vi "ModelParameters.SetModelParameterValue.vi"(8 "Value to Set":dbl, 9 "Channel Name":string, 10 "Target Name":string, 11 "GatewayIP":string) -> (0 "error out":errorcluster)   [LabVIEW 2013, in "MiscHelperVIs.lvlib"]
uses:
  MiscHelperVIs.lvlib
  <vilib>/NI Veristand/Execution/ModelManager/NI VeriStand - Set Single Parameter Value.vi
  <vilib>/NI Veristand/Execution/ModelManager/NI VeriStand - Get Single Parameter Value.vi
  <vilib>/NI Veristand/Execution/ModelManager/NI_VS ModelManager ExecutionAPI.lvlib
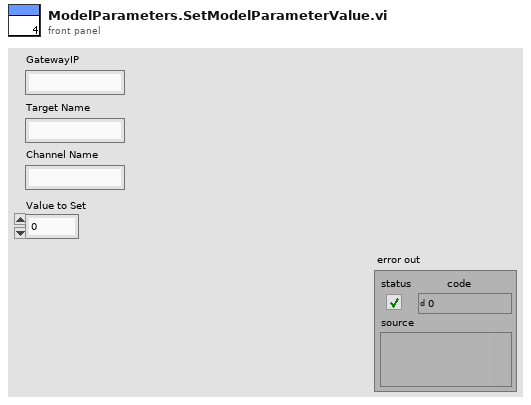
[diagram p1: front panel]
types:
  T1 = typedef "NI_VS ModelManager ExecutionAPI.lvlib/ModelManagerAPI.ctl" = refnum<k24>
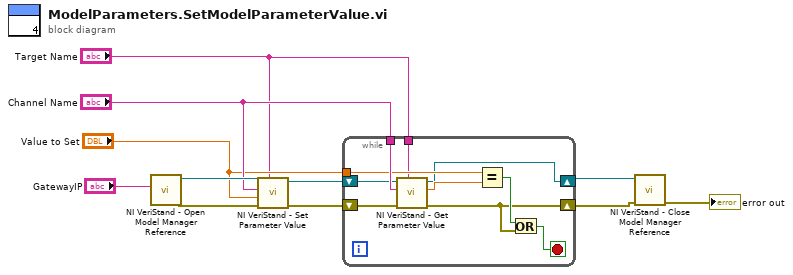
[diagram p0: block diagram]
diagram:
  n1 = call <vilib>:"NI VeriStand - Open Model Manager Reference.vi"("Gateway IP Address (\"\": localhost)"="GatewayIP") -> ("error out"=w10:errorcluster, "ModelManager"=w9:T1)  [unwired: 9 in]
  n2 = call-poly <vilib>:"NI VeriStand - Set Parameter Value.vi"("Target"="Target Name", "error in (no error)"=w10, "Value"="Value to Set", "Parameter"="Channel Name", "ModelManager in"=w9) -> ("error out"=w5:errorcluster, "ModelManager out"=w4:T1)  [unwired: 5 in]
  n3 = while {
    tunnel: "Channel Name" -> [w21]
    tunnel: "Value to Set" -> [w19]
    shift-right: [w14] -> w2
    shift-left: w4 -> [w17]
    tunnel: "Target Name" -> [w13]
    shift-right: [w12] -> w1
    shift-left: w5 -> [w18]
    stop <- w15 stop-if-true
    n4 = call-poly <vilib>:"NI VeriStand - Get Parameter Value.vi"("Target"=w13, "error in (no error)"=w18, "Parameter"=w21, "ModelManager in"=w17) -> ("error out"=w12:errorcluster, "Value"=w20:dbl, "ModelManager out"=w14:T1)  [unwired: 5 in]
    n5 = Equal?(x=w19, y=w20) -> (x = y?=w16:bool)
    n6 = Or(x=w16, y=w12) -> (x .or. y?=w15:bool)
  }
  n7 = call <vilib>:"NI VeriStand - Close Model Manager Reference.vi"("error in (no error)"=w1, "ModelManager"=w2) -> ("error out"=→"error out":errorcluster)  [unwired: 9 in]
